vi "log analysis_gps.vi"() -> ()   [LabVIEW 2019] (continued)
22.3000,0.3276,0.3265,-0.0468,0.306680390,-0.455879554,38.607757832,0.4139,0.2956,0.5455,0.1116,0.0928,0.0789,0.2623,0.2370,5.2072,0f000001,0*4613d5e8\n\tsystem status\tnormal 2 28.100000 0 0\trobot status\t86.793506\t114.356384\t7.882400\t0.306680\t-0.455880\t51.392242\t0.481000\t-0.082000\n\t\n15:10:34.9\tlog_raw\tgps_raw\t#INSPVAXA,USB3,0,44.5,FINESTEERING,2107,281452.900,02000000,471d,15824;INS_ALIGNMENT_COMPLETE,INS_RTKFIXED,37.37116210966,126.72181674670,7.8822,22.3000,0.3215,0.3514,-0.0183,0.377751174,-0.234093113,39.308354629,0.4139,0.2956,0.5455,0.1116,0.0928,0.0789,0.2623,0.2370,5.2072,0f000001,0*f7d4e910\n\tsystem status\tnormal 2 28.100000 0 0\trobot status\t86.952206\t114.526018\t7.882200\t0.377751\t-0.234093\t50.691645\t0.575000\t0.082000\n\t\n15:10:35.4\tlog_raw\tgps_raw\t#INSPVAXA,USB3,0,49.0,FINESTEERING,2107,281453.400,02000000,471d,15824;INS_ALIGNMENT_COMPLETE,INS_RTKFIXED,37.37116361961,126.72181857489,7.8793,22.3000,0.3370,0.3634,-0.0294,0.431370913,-0.173130172,39.969478281,0.4147,0.2957,0.5475,0.1117,0.0928,0.0786,0.2622,0.2369,5.2083,0f000001,0*84da0b27\n\tsystem status\tnormal 2 28.100000 0 0\trobot status\t87.114144\t114.693597\t7.879300\t0.431371\t-0.173130\t50.030522\t0.697000\t0.271000\n\t\n15:10:35.9\tlog_raw\tgps_raw\t#INSPVAXA,USB3,0,49.0,FINESTEERING,2107,281453.900,02000000,471d,15824;INS_ALIGNMENT_COMPLETE,INS_RTKFIXED,37.37116508071,126.72182041170,7.8755,22.3000,0.3222,0.3708,0.0001,0.426257094,0.020843514,40.660737153,0.4147,0.2957,0.5475,0.1117,0.0928,0.0786,0.2622,0.2369,5.2083,0f000001,0*b9aa4650\n\tsystem status\tnormal 2 28.100000 0 0\trobot status\t87.276845\t114.855755\t7.875500\t0.426257\t0.020844\t49.339263\t0.637000\t0.224000\n\t\n15:10:36.4\tlog_raw\tgps_raw\t\tsystem status\tnormal 2 28.200000 0 0\trobot status\t87.425316\t115.004204\t7.873100\t0.306924\t-0.091173\t48.845827\t0.512000\t0.015000\n\t\n15:10:36.9\tlog_raw\tgps_raw\t\tsystem status\tnormal 2 28.200000 0 0\trobot status\t87.594195\t115.169671\t7.870000\t0.055982\t-0.430690\t48.471662\t0.488000\t0.000000\n\t\n15:10:37.4\tlog_raw\tgps_raw\t#INSPVAXA,USB3,0,47.5,FINESTEERING,2107,281455.400,02000000,471d,15824;INS_ALIGNMENT_COMPLETE,INS_RTKFIXED,37.37116944200,126.72182606901,7.8692,22.3000,0.2987,0.3736,-0.0088,0.240749777,-0.612888046,41.923306200,0.4162,0.2974,0.5511,0.1132,0.0944,0.0792,0.2618,0.2366,5.2086,0f000001,0*c27b5d3d\n\tsystem status\tnormal 2 28.200000 0 0\trobot status\t87.777961\t115.339786\t7.869200\t0.240750\t-0.612888\t48.076694\t0.495000\t0.000000\n\t\n15:10:37.9\tlog_raw\tgps_raw\t\tsystem status\tnormal 2 28.200000 0 0\trobot status\t87.930313\t115.479170\t7.868600\t0.020179\t-0.354766\t47.828050\t0.494000\t0.009000\n\t\n15:10:38.4\tlog_raw\tgps_raw\t\tsystem status\tnormal 2 28.200000 0 0\trobot status\t88.096784\t115.631090\t7.865500\t0.013870\t-0.069360\t47.540904\t0.491000\t0.018000\n\t\n15:10:38.9\tlog_raw\tgps_raw\t#INSPVAXA,USB3,0,48.0,FINESTEERING,2107,281456.900,02000000,471d,15824;INS_ALIGNMENT_COMPLETE,INS_RTKFIXED,37.37117357948,126.72183178358,7.8608,22.3000,0.3100,0.3922,-0.0117,-0.041780079,0.015103018,42.742184550,0.4159,0.2958,0.5494,0.1140,0.0949,0.0793,0.2613,0.2363,5.2090,0f000001,0*a764cc08\n\tsystem status\tnormal 2 28.200000 0 0\trobot status\t88.284148\t115.798978\t7.860800\t-0.041780\t0.015103\t47.257815\t0.495000\t0.022000\n\t\n15:10:39.4\tlog_raw\tgps_raw\t\tsystem status\tnormal 2 28.200000 0 0\trobot status\t88.440316\t115.946391\t7.860500\t-0.480884\t-0.081727\t47.108768\t0.484000\t0.025000\n\t\n15:10:39.9\tlog_raw\tgps_raw\t#INSPVAXA,USB3,0,47.5,FINESTEERING,2107,281457.900,02008000,471d,15824;INS_ALIGNMENT_COMPLETE,INS_RTKFIXED,37.37117644696,126.72183567344,7.8614,22.3000,0.3036,0.3952,-0.0191,-0.435122492,0.297928497,42.865174724,0.4156,0.2944,0.5469,0.1149,0.0954,0.0797,0.2607,0.2357,5.2097,0f000001,0*67fee73b\n\tsystem status\tnormal 2 28.200000 0 0\trobot status\t88.628705\t116.117220\t7.861400\t-0.435122\t0.297928\t47.134825\t0.508000\t0.013000\n\t\n15:10:40.4\tlog_raw\tgps_raw\t#INSPVAXA,USB3,0,48.0,FINESTEERING,2107,281458.400,02008000,471d,15824;INS_ALIGNMENT_COMPLETE,INS_RTKFIXED,37.37117789762,126.72183765812,7.8605,22.3000,0.2663,0.3794,0.0055,-0.186627591,0.430628544,42.799150387,0.4156,0.2930,0.5449,0.1157,0.0959,0.0801,0.2599,0.2351,5.2111,0f000001,0*353aab58\n\tsystem status\tnormal 2 28.200000 0 0\trobot status\t88.804505\t116.278219\t7.860500\t-0.186628\t0.430629\t47.200850\t0.465000\t0.064000\n\t\n15:10:40.9\tlog_raw\tgps_raw\t#INSPVAXA,USB3,0,48.0,FINESTEERING,2107,281458.900,02008000,471d,15824;INS_ALIGNMENT_COMPLETE,INS_RTKFIXED,37.37117931784,126.72183956069,7.8626,22.3000,0.2674,0.3686,0.0176,-0.645699086,0.378450815,42.391957050,0.4156,0.2930,0.5449,0.1157,0.0959,0.0801,0.2599,0.2351,5.2111,0f000001,0*1d8f7f17\n\tsystem status\tnormal 2 28.100000 0 0\trobot status\t88.973032\t116.435840\t7.862600\t-0.645699\t0.378451\t47.608043\t0.448000\t0.077000\n\t\n15:10:41.4\tlog_raw\tgps_raw\t\tsystem status\tnormal 2 28.000000 0 0\trobot status\t89.126711\t116.583855\t7.864100\t-0.650969\t0.083856\t48.244986\t0.484000\t0.043000\n\t\n15:10:41.9\tlog_raw\tgps_raw\t#INSPVAXA,USB3,0,50.5,FINESTEERING,2107,281459.900,02008000,471d,15824;INS_ALIGNMENT_COMPLETE,INS_RTKFIXED,37.37118223269,126.72184333763,7.8658,22.3000,0.2701,0.3610,0.0161,-0.453997018,0.223797272,40.778453294,0.4167,0.2944,0.5456,0.1164,0.0966,0.0809,0.2589,0.2343,5.2128,0f000001,0*32172057\n\tsystem status\tnormal 2 28.000000 0 0\trobot status\t89.307587\t116.759340\t7.865800\t-0.453997\t0.223797\t49.221547\t0.809000\t-0.455000\n\t\n15:10:42.4\tlog_raw\tgps_raw\t\tsystem status\tnormal 2 27.900000 0 0\trobot status\t89.451971\t116.913610\t7.868000\t-0.666596\t0.065651\t50.162265\t0.449000\t0.123000\n\t\n15:10:42.9\tlog_raw\tgps_raw\t\tsystem status\tnormal 2 28.000000 0 0\trobot status\t89.609230\t117.086793\t7.867300\t-0.761616\t0.035523\t51.116930\t0.518000\t0.000000\n\t\n15:10:43.4\tlog_raw\tgps_raw\t#INSPVAXA,USB3,0,46.5,FINESTEERING,2107,281461.400,02008000,471d,15824;INS_ALIGNMENT_COMPLETE,INS_RTKFIXED,37.37118692248,126.72184864093,7.8697,22.3000,0.3068,0.3589,-0.0063,-0.709550175,-0.051664009,37.872013250,0.4180,0.2946,0.5458,0.1159,0.0960,0.0825,0.2566,0.2324,5.2151,0f000001,0*59364c44\n\tsystem status\tnormal 2 27.900000 0 0\trobot status\t89.777344\t117.279829\t7.869700\t-0.709550\t-0.051664\t52.127987\t0.587000\t-0.105000\n\t\n15:10:43.9\tlog_raw\tgps_raw\t#INSPVAXA,USB3,0,46.5,FINESTEERING,2107,281461.900,02008000,471d,15824;INS_ALIGNMENT_COMPLETE,INS_RTKFIXED,37.37118851997,126.72185034796,7.8716,22.3000,0.2953,0.3443,0.0004,-0.635296762,0.077766272,37.199284796,0.4180,0.2946,0.5458,0.1159,0.0960,0.0825,0.2566,0.2324,5.2151,0f000001,0*e7cf6597\n\tsystem status\tnormal 2 28.100000 0 0\trobot status\t89.928550\t117.457124\t7.871600\t-0.635297\t0.077766\t52.800715\t0.554000\t-0.077000\n\t\n15:10:44.4\tlog_raw\tgps_raw\t#INSPVAXA,USB3,0,48.0,FINESTEERING,2107,281462.400,02008000,471d,15824;INS_ALIGNMENT_COMPLETE,INS_RTKFIXED,37.37119016469,126.72185198950,7.8718,22.3000,0.3140,0.3274,-0.0278,-0.753643784,0.303209826,36.783589938,0.4170,0.2921,0.5431,0.1150,0.0951,0.0832,0.2556,0.2316,5.2152,0f000001,0*71cc871c\n\tsystem status\tnormal 2 28.100000 0 0\trobot status\t90.073955\t117.639662\t7.871800\t-0.753644\t0.303210\t53.216410\t0.455000\t0.077000\n\t\n15:10:44.9\tlog_raw\tgps_raw\t#INSPVAXA,USB3,0,48.0,FINESTEERING,2107,281462.900,02008000,471d,15824;INS_ALIGNMENT_COMPLETE,INS_RTKFIXED,37.37119183431,126.72185366937,7.8730,22.3000,0.3211,0.3220,0.0114,-0.696465200,0.281664462,36.480823523,0.4170,0.2921,0.5431,0.1150,0.0951,0.0832,0.2556,0.2316,5.2152,0f000001,0*b2de4003\n\tsystem status\tnormal 2 28.100000 0 0\trobot status\t90.222755\t117.824962\t7.873000\t-0.696465\t0.281664\t53.519176\t0.660000\t-0.248000\n\t\n15:10:45.4\tlog_raw\tgps_raw\t#INSPVAXA,USB3,0,48.5,FINESTEERING,2107,281463.400,02008000,471d,15824;INS_ALIGNMENT_COMPLETE,INS_RTKFIXED,37.37119351156,126.72185532212,7.8740,22.3000,0.2696,0.3105,-0.0010,-0.845084934,0.040994289,36.443862142,0.4171,0.2926,0.5444,0.1146,0.0951,0.0842,0.2547,0.2310,5.2149,0f000001,0*1ae650cc\n\tsystem status\tnormal 2 28.100000 0 0\trobot status\t90.369153\t118.011109\t7.874000\t-0.845085\t0.040994\t53.556138\t0.360000\t0.131000\n\t\n15:10:45.9\tlog_raw\tgps_raw\t#INSPVAXA,USB3,0,48.5,FINESTEERING,2107,281463.900,02008000,471d,15824;INS_ALIGNMENT_COMPLETE,INS_RTKFIXED,37.37119483302,126.72185668642,7.8760,22.3000,0.1153,0.1917,-0.0076,-0.816856486,-0.145545038,36.378444891,0.4171,0.2926,0.5444,0.1146,0.0951,0.0842,0.2547,0.2310,5.2149,0f000001,0*1c1cdd38\n\tsystem status\tnormal 2 28.200000 0 0\trobot status\t90.490001\t118.157770\t7.876000\t-0.816856\t-0.145545\t53.621555\t0.368000\t-0.116000\n\t\n15:10:46.4\tlog_raw\tgps_raw\t#INSPVAXA,USB3,0,45.5,FINESTEERING,2107,281464.400,02000000,471d,15824;INS_ALIGNMENT_COMPLETE,INS_RTKFIXED,37.37119579175,126.72185768591,7.8792,22.3000,0.1971,0.2398,0.0010,-0.742386203,-0.127943073,36.538622941,0.4195,0.2979,0.5527,0.1161,0.0973,0.0858,0.2541,0.2308,5.2143,0f000001,0*24dc1fe0\n\tsystem status\tnormal 2 28.200000 0 0\trobot status\t90.578534\t118.264173\t7.879200\t-0.742386\t-0.127943\t53.461377\t0.317000\t-0.011000\n\t\n15:10:46.9\tlog_raw\tgps_raw\t#INSPVAXA,USB3,0,45.5,FINESTEERING,2107,281464.900,02000000,471d,15824;INS_ALIGNMENT_COMPLETE,INS_RTKFIXED,37.37119672915,126.72185869204,7.8846,22.3000,0.1715,0.2230,-0.0041,-0.675547372,-0.136073790,36.631506264,0.4195,0.2979,0.5527,0.1161,0.0973,0.0858,0.2541,0.2308,5.2143,0f000001,0*e856a3ba\n\tsystem status\tnormal 2 28.200000 0 0\trobot status\t90.667655\t118.368209\t7.884600\t-0.675547\t-0.136074\t53.368494\t0.292000\t-0.024000\n\t\n15:10:47.4\tlog_raw\tgps_raw\t#INSPVAXA,USB3,0,49.0,FINESTEERING,2107,281465.400,02000000,471d,15824;INS_ALIGNMENT_COMPLETE,INS_RTKFIXED,37.37119777976,126.72185974580,7.8895,22.3000,0.1707,0.2152,-0.0021,-0.795130387,-0.134235456,36.862190913,0.4216,0.3036,0.5603,0.1136,0.0955,0.0851,0.2538,0.2307,5.2127,0f000001,0*3dceb74e\n\tsystem status\tnormal 2 28.200000 0 0\trobot status\t90.760996\t118.484810\t7.889500\t-0.795130\t-0.134235\t53.137809\t0.295000\t-0.028000\n\t\n15:10:47.9\tlog_raw\tgps_raw\t#INSPVAXA,USB3,0,49.0,FINESTEERING,2107,281465.900,02000000,471d,15824;INS_ALIGNMENT_COMPLETE,INS_RTKFIXED,37.37119882408,126.72186080871,7.8935,22.3000,0.1975,0.2377,-0.0103,-0.927101285,0.026313679,37.093891060,0.4216,0.3036,0.5603,0.1136,0.0955,0.0851,0.2538,0.2307,5.2127,0f000001,0*b32abc1e\n\tsystem status\tnormal 2 28.200000 0 0\trobot status\t90.855146\t118.600712\t7.893500\t-0.927101\t0.026314\t52.906109\t0.296000\t-0.025000\n\t\n15:10:48.4\tlog_raw\tgps_raw\t#INSPVAXA,USB3,0,45.5,FINESTEERING,2107,281466.400,02000000,471d,15824;INS_ALIGNMENT_COMPLETE,INS_RTKFIXED,37.37119994764,126.72186191360,7.8953,22.3000,0.1896,0.2516,0.0024,-0.990040985,-0.050764765,37.290261699,0.4218,0.3053,0.5656,0.1126,0.0944,0.0842,0.2536,0.2306,5.2108,0f000001,0*ab7ec7da\n\tsystem status\tnormal 2 28.200000 0 0\trobot status\t90.953016\t118.725409\t7.895300\t-0.990041\t-0.050765\t52.709738\t0.299000\t-0.020000\n\t\n15:10:48.9\tlog_raw\tgps_raw\t#INSPVAXA,USB3,0,45.5,FINESTEERING,2107,281466.900,02000000,471d,15824;INS_ALIGNMENT_COMPLETE,INS_RTKFIXED,37.37120100149,126.72186298872,7.8973,22.3000,0.1935,0.2522,-0.0026,-0.854741520,-0.119099122,37.564308734,0.4218,0.3053,0.5656,0.1126,0.0944,0.0842,0.2536,0.2306,5.2108,0f000001,0*b7c581e3\n\tsystem status\tnormal 2 28.200000 0 0\trobot status\t91.048248\t118.842369\t7.897300\t-0.854742\t-0.119099\t52.435691\t0.315000\t-0.002000\n\t\n15:10:49.4\tlog_raw\tgps_raw\t#INSPVAXA,USB3,0,48.0,FINESTEERING,2107,281467.400,02000000,471d,15824;INS_ALIGNMENT_COMPLETE,INS_RTKFIXED,37.37120208153,126.72186408522,7.8997,22.3000,0.1778,0.2253,0.0049,-0.719912945,-0.270478243,38.035475922,0.4244,0.3113,0.5828,0.1121,0.0950,0.0843,0.2538,0.2306,5.2092,0f000001,0*8e9732d5\n\tsystem status\tnormal 2 28.200000 0 0\trobot status\t91.145374\t118.962236\t7.899700\t-0.719913\t-0.270478\t51.964524\t0.217000\t-0.146000\n\t\n15:10:49.9\tlog_raw\tgps_raw\t#INSPVAXA,USB3,0,48.0,FINESTEERING,2107,281467.900,02000000,471d,15824;INS_ALIGNMENT_COMPLETE,INS_RTKFIXED,37.37120312889,126.72186517178,7.9031,22.3000,0.2039,0.2426,0.0147,-0.720629061,-0.231870268,38.725653809,0.4244,0.3113,0.5828,0.1121,0.0950,0.0843,0.2538,0.2306,5.2092,0f000001,0*c758e7ce\n\tsystem status\tnormal 2 28.100000 0 0\trobot status\t91.241620\t119.078476\t7.903100\t-0.720629\t-0.231870\t51.274346\t0.251000\t-0.107000\n\t\n15:10:50.4\tlog_raw\tgps_raw\t#INSPVAXA,USB3,0,48.5,FINESTEERING,2107,281468.400,02000000,471d,15824;INS_ALIGNMENT_COMPLETE,INS_RTKFIXED,37.37120416086,126.72186625746,7.9066,22.3000,0.2025,0.2267,-0.0001,-0.736489084,-0.165649528,39.721937458,0.4260,0.3144,0.5975,0.1120,0.0953,0.0842,0.2539,0.2306,5.2089,0f000001,0*64b5bba4\n\tsystem status\tnormal 2 28.000000 0 0\trobot status\t91.337788\t119.193007\t7.906600\t-0.736489\t-0.165650\t50.278063\t0.273000\t-0.077000\n\t\n15:10:50.9\tlog_raw\tgps_raw\t#INSPVAXA,USB3,0,48.5,FINESTEERING,2107,281468.900,02000000,471d,15824;INS_ALIGNMENT_COMPLETE,INS_RTKFIXED,37.37120515414,126.72186733248,7.9096,22.3000,0.1860,0.2130,0.0062,-0.863833957,-0.176893088,40.861857992,0.4260,0.3144,0.5975,0.1120,0.0953,0.0842,0.2539,0.2306,5.2089,0f000001,0*48502021\n\tsystem status\tnormal 2 28.000000 0 0\trobot status\t91.433011\t119.303245\t7.909600\t-0.863834\t-0.176893\t49.138142\t0.282000\t-0.055000\n\t\n15:10:51.4\tlog_raw\tgps_raw\t#INSPVAXA,USB3,0,47.5,FINESTEERING,2107,281469.400,02000000,471d,15824;INS_ALIGNMENT_COMPLETE,INS_RTKFIXED,37.37120615783,126.72186845955,7.9127,22.3000,0.1833,0.2266,0.0157,-0.922756560,-0.128393101,41.953959499,0.4267,0.3157,0.6087,0.1119,0.0952,0.0838,0.2539,0.2306,5.2092,0f000001,0*9d6cc6cc\n\tsystem status\tnormal 2 28.000000 0 0\trobot status\t91.532845\t119.414638\t7.912700\t-0.922757\t-0.128393\t48.046041\t0.232000\t-0.142000\n\t\n15:10:51.9\tlog_raw\tgps_raw\t#INSPVAXA,USB3,0,47.5,FINESTEERING,2107,281469.900,02000000,471d,15824;INS_ALIGNMENT_COMPLETE,INS_RTKFIXED,37.37120711333,126.72186961218,7.9172,22.3000,0.1882,0.2386,0.0103,-0.812681162,-0.149481379,43.058831500,0.4267,0.3157,0.6087,0.1119,0.0952,0.0838,0.2539,0.2306,5.2092,0f000001,0*7e42c462\n\tsystem status\tnormal 2 28.000000 0 0\trobot status\t91.634943\t119.520683\t7.917200\t-0.812681\t-0.149481\t46.941169\t0.239000\t-0.134000\n\t\n15:10:52.4\tlog_raw\tgps_raw\t#INSPVAXA,USB3,0,48.0,FINESTEERING,2107,281470.400,02000000,471d,15824;INS_ALIGNMENT_COMPLETE,INS_RTKFIXED,37.37120802040,126.72187075599,7.9242,22.3000,0.1759,0.2315,0.0092,-0.712389099,-0.099720322,44.115258492,0.4228,0.3076,0.5975,0.1114,0.0938,0.0818,0.2538,0.2305,5.2102,0f000001,0*4e20fbfc\n\tsystem status\tnormal 2 28.000000 0 0\trobot status\t91.736260\t119.621353\t7.924200\t-0.712389\t-0.099720\t45.884742\t0.231000\t-0.116000\n\t\n15:10:52.9\tlog_raw\tgps_raw\t#INSPVAXA,USB3,0,48.0,FINESTEERING,2107,281470.900,02000000,471d,15824;INS_ALIGNMENT_COMPLETE,INS_RTKFIXED,37.37120891997,126.72187193685,7.9313,22.3000,0.1721,0.2325,0.0046,-0.682625247,-0.034958907,44.921832107,0.4228,0.3076,0.5975,0.1114,0.0938,0.0818,0.2538,0.2305,5.2102,0f000001,0*8a1ed08d\n\tsystem status\tnormal 2 28.100000 0 0\trobot status\t91.840859\t119.721190\t7.931300\t-0.682625\t-0.034959\t45.078168\t0.251000\t-0.082000\n\t\n15:10:53.4\tlog_raw\tgps_raw\t#INSPVAXA,USB3,0,44.5,FINESTEERING,2107,281471.400,02000000,471d,15824;INS_ALIGNMENT_COMPLETE,INS_RTKFIXED,37.37120978762,126.72187309291,7.9372,22.3000,0.1737,0.2402,0.0107,-0.896905071,0.182357572,45.734122702,0.4207,0.3039,0.5902,0.1115,0.0938,0.0806,0.2537,0.2305,5.2115,0f000001,0*f5531b04\n\tsystem status\tnormal 2 28.100000 0 0\trobot status\t91.943261\t119.817484\t7.937200\t-0.896905\t0.182358\t44.265877\t0.307000\t0.000000\n\t\n15:10:53.9\tlog_raw\tgps_raw\t#DUALANTENNAHEADINGA,USB3,0,44.5,FINESTEERING,2107,281471.900,02000000,d426,15824;SOL_COMPUTED,NARROW_FLOAT,-1.000000000,14.722629547,3.656694651,0.0,237.736404419,180.000000000,\"631T\",22,8,8,7,04,00,20,03*d908accb\n\tsystem status\tnormal 2 28.100000 0 0\trobot status\t92.048574\t119.910495\t7.943000\t-0.828598\t0.376591\t43.556063\t0.292000\t-0.018000\n\t\n15:10:54.4\tlog_raw\tgps_raw\t#INSPVAXA,USB3,0,44.5,FINESTEERING,2107,281472.400,02000000,471d,15824;INS_ALIGNMENT_COMPLETE,INS_RTKFIXED,37.37121145223,126.72187546991,7.9481,22.3000,0.1558,0.2299,0.0072,-0.729574410,0.299435928,46.987178524,0.4186,0.2997,0.5808,0.1119,0.0940,0.0794,0.2536,0.2304,5.2130,0f000001,0*ceccfdc7\n\tsystem status\tnormal 2 28.100000 0 0\trobot status\t92.153812\t120.002228\t7.948100\t-0.729574\t0.299436\t43.012821\t0.260000\t-0.072000\n\t\n15:10:54.9\tlog_raw\tgps_raw\t#DUALANTENNAHEADINGA,USB3,0,44.5,FINESTEERING,2107,281472.900,02000000,d426,15824;SOL_COMPUTED,NARROW_FLOAT,-1.000000000,19.887695313,3.310185432,0.0,262.944793701,180.000000000,\"631T\",19,8,8,7,04,00,20,03*e2f42a0a\n\tsystem status\tnormal 2 28.200000 0 0\trobot status\t92.259933\t120.093905\t7.952900\t-0.809538\t0.257343\t42.590447\t0.214000\t-0.135000\n\t\n15:10:55.4\tlog_raw\tgps_raw\t#INSPVAXA,USB3,0,47.0,FINESTEERING,2107,281473.400,02000000,471d,15824;INS_ALIGNMENT_COMPLETE,INS_RTKFIXED,37.37121309194,126.72187787297,7.9563,22.3000,0.1608,0.2402,-0.0008,-0.731141510,0.324719411,47.702294704,0.4170,0.2975,0.5726,0.1126,0.0945,0.0786,0.2534,0.2303,5.2142,0f000001,0*03d357e2\n\tsystem status\tnormal 2 28.200000 0 0\trobot status\t92.366671\t120.184208\t7.956300\t-0.731142\t0.324719\t42.297705\t0.287000\t-0.020000\n\t\n15:10:55.9\tlog_raw\tgps_raw\t#INSPVAXA,USB3,0,47.0,FINESTEERING,2107,281473.900,02000000,471d,15824;INS_ALIGNMENT_COMPLETE,INS_RTKFIXED,37.37121388735,126.72187905524,7.9593,22.3000,0.1511,0.2341,0.0050,-0.781655169,0.200652129,47.998434662,0.4170,0.2975,0.5726,0.1126,0.0945,0.0786,0.2534,0.2303,5.2142,0f000001,0*3307b87f\n\tsystem status\tnormal 2 28.200000 0 0\trobot status\t92.471394\t120.272486\t7.959300\t-0.781655\t0.200652\t42.001565\t0.293000\t-0.007000\n\t\n15:10:56.4\tlog_raw\tgps_raw\t#INSPVAXA,USB3,0,50.0,FINESTEERING,2107,281474.400,02000000,471d,15824;INS_ALIGNMENT_COMPLETE,INS_RTKFIXED,37.37121466825,126.72188022113,7.9625,22.3000,0.1592,0.2409,0.0043,-0.925136185,0.519912466,48.197361455,0.4159,0.2959,0.5651,0.1133,0.0951,0.0780,0.2531,0.2301,5.2153,0f000001,0*acbf0539\n\tsystem status\tnormal 2 28.200000 0 0\trobot status\t92.574667\t120.359152\t7.962500\t-0.925136\t0.519912\t41.802639\t0.302000\t0.000000\n\t\n15:10:56.9\tlog_raw\tgps_raw\t#DUALANTENNAHEADINGA,USB3,0,50.0,FINESTEERING,2107,281474.900,02000000,d426,15824;SOL_COMPUTED,L1_FLOAT,-1.000000000,29.703872681,-19.285949707,0.0,227.925506592,180.000000000,\"631T\",19,7,7,7,04,00,20,02*438e8014\n\tsystem status\tnormal 2 28.200000 0 0\trobot status\t92.679329\t120.444310\t7.964600\t-1.008820\t0.706696\t41.621049\t0.299000\t0.004000\n\t\n15:10:57.4\tlog_raw\tgps_raw\t#INSPVAXA,USB3,0,48.0,FINESTEERING,2107,281475.400,02000000,471d,15824;INS_ALIGNMENT_COMPLETE,INS_RTKFIXED,37.37121622258,126.72188269700,7.9646,22.3000,0.1441,0.2253,0.0054,-0.653688748,0.578968322,48.454145381,0.4152,0.2943,0.5583,0.1140,0.0955,0.0776,0.2526,0.2297,5.2166,0f000001,0*7e585380\n\tsystem status\tnormal 2 28.200000 0 0\trobot status\t92.793975\t120.531657\t7.964600\t-0.653689\t0.578968\t41.545855\t0.300000\t0.000000\n\t\n15:10:57.9\tlog_raw\tgps_raw\t#INSPVAXA,USB3,0,48.0,FINESTEERING,2107,281475.900,02000000,471d,15824;INS_ALIGNMENT_COMPLETE,INS_RTKFIXED,37.37121692154,126.72188386600,7.9655,22.3000,0.1584,0.2123,0.0124,-0.619737810,0.551987551,48.617638369,0.4152,0.2943,0.5583,0.1140,0.0955,0.0776,0.2526,0.2297,5.2166,0f000001,0*cdba2d64\n\tsystem status\tnormal 2 28.200000 0 0\trobot status\t92.897523\t120.609229\t7.965500\t-0.619738\t0.551988\t41.382362\t0.301000\t0.002000\n\t\n15:10:58.4\tlog_raw\tgps_raw\t#INSPVAXA,USB3,0,46.5,FINESTEERING,2107,281476.400,02000000,471d,15824;INS_ALIGNMENT_COMPLETE,INS_RTKFIXED,37.37121768155,126.72188507525,7.9668,22.3000,0.1354,0.2014,0.0180,-0.822035432,0.378941407,48.791141972,0.4147,0.2931,0.5519,0.1146,0.0957,0.0772,0.2519,0.2292,5.2180,0f000001,0*1e1562b5\n\tsystem status\tnormal 2 28.200000 0 0\trobot status\t93.004637\t120.693577\t7.966800\t-0.822035\t0.378941\t41.208858\t0.292000\t0.001000\n\t\n15:10:58.9\tlog_raw\tgps_raw\t#INSPVAXA,USB3,0,46.5,FINESTEERING,2107,281476.900,02000000,471d,15824;INS_ALIGNMENT_COMPLETE,INS_RTKFIXED,37.37121850161,126.72188636358,7.9688,22.3000,0.1738,0.2367,0.0108,-1.201696541,-0.232647671,48.968391321,0.4147,0.2931,0.5519,0.1146,0.0957,0.0772,0.2519,0.2292,5.2180,0f000001,0*afd5e89e\n\tsystem status\tnormal 2 28.200000 0 0\trobot status\t93.118755\t120.784590\t7.968800\t-1.201697\t-0.232648\t41.031609\t0.304000\t0.013000\n\t\n15:10:59.4\tlog_raw\tgps_raw\t#INSPVAXA,USB3,0,50.5,FINESTEERING,2107,281477.400,02000000,471d,15824;INS_ALIGNMENT_COMPLETE,INS_RTKFIXED,37.37121929078,126.72188763502,7.9707,22.3000,0.1401,0.2321,0.0104,-1.230903565,-0.339648847,49.051409136,0.4145,0.2921,0.5464,0.1152,0.0963,0.0770,0.2510,0.2285,5.2193,0f000001,0*fd6eca37\n\tsystem status\tnormal 2 28.200000 0 0\trobot status\t93.231377\t120.872175\t7.970700\t-1.230904\t-0.339649\t40.948591\t0.304000\t0.018000\n\t\n15:10:59.9\tlog_raw\tgps_raw\t#DUALANTENNAHEADINGA,USB3,0,50.5,FINESTEERING,2107,281477.900,02000000,d426,15824;SOL_COMPUTED,NARROW_FLOAT,-1.000000000,24.973518372,-6.230041504,0.0,279.644378662,180.000000000,\"631T\",18,8,8,6,04,00,20,03*2ec7f676\n\tsystem status\tnormal 2 28.200000 0 0\trobot status\t93.343059\t120.954830\t7.971600\t-1.076063\t-0.162518\t40.856489\t0.301000\t0.004000\n\t\n15:11:00.4\tlog_raw\tgps_raw\t#DUALANTENNAHEADINGA,USB3,0,45.5,FINESTEERING,2107,281478.400,02000000,d426,15824;SOL_COMPUTED,NARROW_FLOAT,-1.000000000,25.984382629,-14.421966553,0.0,321.839630127,180.000000000,\"631T\",19,7,7,6,04,00,20,03*c537a035\n\tsystem status\tnormal 2 28.200000 0 0\trobot status\t93.457296\t121.042717\t7.970400\t-1.082595\t-0.386242\t40.815336\t0.306000\t0.000000\n\t\n15:11:00.9\tlog_raw\tgps_raw\t#INSPVAXA,USB3,0,45.5,FINESTEERING,2107,281478.900,02000000,471d,15824;INS_ALIGNMENT_COMPLETE,INS_RTKFIXED,37.37122160716,126.72189152509,7.9681,22.3000,0.1537,0.2575,-0.0106,-0.771104700,-0.770425381,49.241520291,0.4142,0.2902,0.5416,0.1154,0.0959,0.0768,0.2499,0.2277,5.2192,0f000001,0*21e6a269\n\tsystem status\tnormal 2 28.200000 0 0\trobot status\t93.575953\t121.129253\t7.968100\t-0.771105\t-0.770425\t40.758480\t0.317000\t-0.004000\n\t\n15:11:01.4\tlog_raw\tgps_raw\t#INSPVAXA,USB3,0,48.0,FINESTEERING,2107,281479.400,02000000,471d,15824;INS_ALIGNMENT_COMPLETE,INS_RTKFIXED,37.37122237259,126.72189283393,7.9651,22.3000,0.1293,0.2257,0.0059,-0.612587772,-1.097823401,49.383599810,0.4139,0.2890,0.5376,0.1159,0.0956,0.0767,0.2487,0.2267,5.2174,0f000001,0*f7632e7f\n\tsystem status\tnormal 2 28.200000 0 0\trobot status\t93.691888\t121.214203\t7.965100\t-0.612588\t-1.097823\t40.616400\t0.292000\t0.007000\n\t\n15:11:01.9\tlog_raw\tgps_raw\t#INSPVAXA,USB3,0,48.0,FINESTEERING,2107,281479.900,02000000,471d,15824;INS_ALIGNMENT_COMPLETE,INS_RTKFIXED,37.37122311792,126.72189412346,7.9647,22.3000,0.1494,0.2660,0.0073,-0.587954124,-1.340332352,49.363469621,0.4139,0.2890,0.5376,0.1159,0.0956,0.0767,0.2487,0.2267,5.2174,0f000001,0*4724fb20\n\tsystem status\tnormal 2 28.200000 0 0\trobot status\t93.806112\t121.296922\t7.964700\t-0.587954\t-1.340332\t40.636530\t0.319000\t-0.007000\n\t\n15:11:02.4\tlog_raw\tgps_raw\t#DUALANTENNAHEADINGA,USB3,0,48.5,FINESTEERING,2107,281480.400,02000000,d426,15824;SOL_COMPUTED,L1_FLOAT,-1.000000000,38.387950897,-13.434600830,0.0,360.000000000,180.000000000,\"631T\",19,7,7,7,04,00,20,02*88d00c71\n\tsystem status\tnormal 2 28.200000 0 0\trobot status\t93.918035\t121.383471\t7.961400\t-0.891588\t-1.356831\t40.747449\t0.284000\t0.019000\n\t\n15:11:02.9\tlog_raw\tgps_raw\t#DUALANTENNAHEADINGA,USB3,0,48.5,FINESTEERING,2107,281480.900,02000000,d426,15824;SOL_COMPUTED,L1_FLOAT,-1.000000000,37.718753815,-13.467346191,0.0,360.000000000,180.000000000,\"631T\",19,7,7,7,04,00,20,02*9128bd3b\n\tsystem status\tnormal 2 28.200000 0 0\trobot status\t94.032799\t121.467213\t7.959200\t-0.622653\t-1.342414\t40.873530\t0.308000\t0.007000\n\t\n15:11:03.4\tlog_raw\tgps_raw\t#DUALANTENNAHEADINGA,USB3,0,46.5,FINESTEERING,2107,281481.400,02008000,d426,15824;SOL_COMPUTED,NARROW_FLOAT,-1.000000000,32.154727936,-10.026550293,0.0,255.698348999,180.000000000,\"631T\",21,8,8,7,04,00,20,03*90654ace\n\tsystem status\tnormal 2 28.200000 0 0\trobot status\t94.141894\t121.548882\t7.956300\t-0.409636\t-0.873487\t41.052834\t0.272000\t0.043000\n\t\n15:11:03.9\tlog_raw\tgps_raw\t#INSPVAXA,USB3,0,46.5,FINESTEERING,2107,281481.900,02008000,471d,15824;INS_ALIGNMENT_COMPLETE,INS_RTKFIXED,37.37122611752,126.72189916270,7.9537,22.3000,0.1376,0.2362,0.0025,-0.095529965,-0.586716272,48.576302995,0.4131,0.2860,0.5308,0.1150,0.0939,0.0764,0.2461,0.2246,5.2038,0f000001,0*d4dc6a04\n\tsystem status\tnormal 2 28.200000 0 0\trobot status\t94.252480\t121.629826\t7.953700\t-0.095530\t-0.586716\t41.423697\t0.320000\t-0.027000\n\t\n15:11:04.4\tlog_raw\tgps_raw\t#INSPVAXA,USB3,0,43.0,FINESTEERING,2107,281482.400,02008000,471d,15824;INS_ALIGNMENT_COMPLETE,INS_RTKFIXED,37.37122693129,126.72190044241,7.9507,22.3000,0.1400,0.2344,0.0009,-0.286718935,-0.542573010,48.417760410,0.4129,0.2856,0.5284,0.1143,0.0930,0.0764,0.2448,0.2237,5.1963,0f000001,0*4b0c873a\n\tsystem status\tnormal 2 28.200000 0 0\trobot status\t94.365835\t121.720141\t7.950700\t-0.286719\t-0.542573\t41.582240\t0.267000\t0.048000\n\t\n15:11:04.9\tlog_raw\tgps_raw\t#DUALANTENNAHEADINGA,USB3,0,43.0,FINESTEERING,2107,281482.900,02008000,d426,15824;SOL_COMPUTED,NARROW_FLOAT,-1.000000000,25.759243011,-24.488281250,0.0,296.027648926,180.000000000,\"631T\",21,7,7,7,04,00,20,03*7949ae50\n\tsystem status\tnormal 2 28.200000 0 0\trobot status\t94.478144\t121.806754\t7.948700\t-0.274138\t-0.373902\t41.735381\t0.350000\t-0.089000\n\t\n15:11:05.4\tlog_raw\tgps_raw\t#DUALANTENNAHEADINGA,USB3,0,49.0,FINESTEERING,2107,281483.400,02008000,d426,15824;SOL_COMPUTED,NARROW_FLOAT,-1.000000000,21.557176590,-28.431182861,0.0,309.766693115,180.000000000,\"631T\",20,8,8,7,04,00,20,03*24e13096\n\tsystem status\tnormal 2 28.200000 0 0\trobot status\t94.589326\t121.896946\t7.946400\t-0.509419\t-0.366117\t41.873006\t0.276000\t0.026000\n\t\n15:11:05.9\tlog_raw\tgps_raw\t#INSPVAXA,USB3,0,49.0,FINESTEERING,2107,281483.900,02008000,471d,15824;INS_ALIGNMENT_COMPLETE,INS_RTKFIXED,37.37122933882,126.72190424641,7.9440,22.3000,0.1298,0.2079,0.0016,-0.555050997,-0.344115137,48.037628133,0.4121,0.2847,0.5256,0.1130,0.0922,0.0763,0.2437,0.2229,5.1908,0f000001,0*4fcd94af\n\tsystem status\tnormal 2 28.200000 0 0\trobot status\t94.702787\t121.987336\t7.944000\t-0.555051\t-0.344115\t41.962372\t0.275000\t0.015000\n\t\n15:11:06.4\tlog_raw\tgps_raw\t#DUALANTENNAHEADINGA,USB3,0,50.0,FINESTEERING,2107,281484.400,02008000,d426,15824;SOL_COMPUTED,L1_FLOAT,-1.000000000,37.365016937,-21.970794678,0.0,360.000000000,180.000000000,\"631T\",19,7,7,7,04,00,20,02*e133e505\n\tsystem status\tnormal 2 28.200000 0 0\trobot status\t94.816092\t122.078802\t7.941300\t-0.509214\t-0.388195\t41.927434\t0.246000\t0.068000\n\t\n15:11:06.9\tlog_raw\tgps_raw\t#INSPVAXA,USB3,0,50.0,FINESTEERING,2107,281484.900,02008000,471d,15824;INS_ALIGNMENT_COMPLETE,INS_RTKFIXED,37.37123096597,126.72190680248,7.9384,22.3000,0.1511,0.2333,-0.0078,-0.410489938,-0.523354884,48.112153719,0.4115,0.2844,0.5237,0.1121,0.0916,0.0762,0.2426,0.2223,5.1884,0f000001,0*a1f40ef1\n\tsystem status\tnormal 2 28.200000 0 0\trobot status\t94.929199\t122.167922\t7.938400\t-0.410490\t-0.523355\t41.887846\t0.307000\t-0.014000\n\t\n15:11:07.4\tlog_raw\tgps_raw\t#DUALANTENNAHEADINGA,USB3,0,47.5,FINESTEERING,2107,281485.400,02000000,d426,15824;SOL_COMPUTED,NARROW_FLOAT,-1.000000000,34.474456787,-26.341827393,0.0,271.964752197,180.000000000,\"631T\",20,7,7,7,04,00,20,03*cc121194\n\tsystem status\tnormal 2 28.200000 0 0\trobot status\t95.038197\t122.255744\t7.935200\t-0.314008\t-0.724193\t41.803910\t0.301000\t-0.018000\n\t\n15:11:07.9\tlog_raw\tgps_raw\t#INSPVAXA,USB3,0,47.5,FINESTEERING,2107,281485.900,02000000,471d,15824;INS_ALIGNMENT_COMPLETE,INS_RTKFIXED,37.37123256957,126.72190927922,7.9317,22.3000,0.1299,0.2173,-0.0089,-0.426845608,-0.944074849,48.432879849,0.4110,0.2838,0.5218,0.1115,0.0911,0.0761,0.2417,0.2218,5.1881,0f000001,0*ee8ace9e\n\tsystem status\tnormal 2 28.200000 0 0\trobot status\t95.148585\t122.345895\t7.931700\t-0.426846\t-0.944075\t41.567120\t0.296000\t-0.027000\n\t\n15:11:08.4\tlog_raw\tgps_raw\t#DUALANTENNAHEADINGA,USB3,0,48.0,FINESTEERING,2107,281486.400,02000000,d426,15824;SOL_COMPUTED,L1_FLOAT,-1.000000000,34.864692688,-21.694915771,0.0,360.000000000,180.000000000,\"631T\",20,7,7,7,04,00,20,02*de044530\n\tsystem status\tnormal 2 28.200000 0 0\trobot status\t95.254925\t122.434334\t7.929200\t-0.583118\t-0.955090\t41.390209\t0.295000\t-0.028000\n\t\n15:11:08.9\tlog_raw\tgps_raw\t#DUALANTENNAHEADINGA,USB3,0,48.0,FINESTEERING,2107,281486.900,02000000,d426,15824;SOL_COMPUTED,L1_FLOAT,-1.000000000,35.417118073,-21.326538086,0.0,360.000000000,180.000000000,\"631T\",20,7,7,7,04,00,20,02*a4d3627b\n\tsystem status\tnormal 2 28.200000 0 0\trobot status\t95.374786\t122.532706\t7.926900\t-0.619494\t-0.937051\t41.183853\t0.303000\t-0.026000\n\t\n15:11:09.4\tlog_raw\tgps_raw\t#INSPVAXA,USB3,0,48.5,FINESTEERING,2107,281487.400,02000000,471d,15824;INS_ALIGNMENT_COMPLETE,INS_RTKFIXED,37.37123510484,126.72191313192,7.9239,22.3000,0.1508,0.2267,-0.0041,-0.710611469,-0.697297129,49.092383754,0.4097,0.2833,0.5200,0.1105,0.0907,0.0760,0.2404,0.2213,5.1897,0f000001,0*65fc2fbf\n\tsystem status\tnormal 2 28.200000 0 0\trobot status\t95.489851\t122.627267\t7.923900\t-0.710611\t-0.697297\t40.907616\t0.238000\t-0.131000\n\t\n15:11:09.9\tlog_raw\tgps_raw\t#INSPVAXA,USB3,0,48.5,FINESTEERING,2107,281487.900,02000000,471d,15824;INS_ALIGNMENT_COMPLETE,INS_RTKFIXED,37.37123588578,126.72191437981,7.9197,22.3000,0.1455,0.2377,-0.0129,-0.683157100,-0.548580830,49.602033608,0.4097,0.2833,0.5200,0.1105,0.0907,0.0760,0.2404,0.2213,5.1897,0f000001,0*fc400f11\n\tsystem status\tnormal 2 28.200000 0 0\trobot status\t95.600387\t122.713938\t7.919700\t-0.683157\t-0.548581\t40.397966\t0.257000\t-0.091000\n\t\n15:11:10.4\tlog_raw\tgps_raw\t#INSPVAXA,USB3,0,47.5,FINESTEERING,2107,281488.400,02000000,471d,15824;INS_ALIGNMENT_COMPLETE,INS_RTKFIXED,37.37123668548,126.72191567046,7.9173,22.3000,0.1286,0.2563,0.0010,-0.700638856,-0.301855154,50.490709534,0.4091,0.2828,0.5195,0.1103,0.0906,0.0760,0.2400,0.2212,5.1909,0f000001,0*20940426\n\tsystem status\tnormal 2 28.000000 0 0\trobot status\t95.714710\t122.802691\t7.917300\t-0.700639\t-0.301855\t39.509290\t0.289000\t-0.057000\n\t\n15:11:10.9\tlog_raw\tgps_raw\t#INSPVAXA,USB3,0,47.5,FINESTEERING,2107,281488.900,02000000,471d,15824;INS_ALIGNMENT_COMPLETE,INS_RTKFIXED,37.37123745255,126.72191698522,7.9152,22.3000,0.1363,0.2513,-0.0110,-0.588840465,-0.298661481,51.824057860,0.4091,0.2828,0.5195,0.1103,0.0906,0.0760,0.2400,0.2212,5.1909,0f000001,0*3253a0a6\n\tsystem status\tnormal 2 28.000000 0 0\trobot status\t95.831170\t122.887822\t7.915200\t-0.588840\t-0.298661\t38.175942\t0.297000\t-0.069000\n\t\n15:11:11.4\tlog_raw\tgps_raw\t#DUALANTENNAHEADINGA,USB3,0,48.5,FINESTEERING,2107,281489.400,02000000,d426,15824;SOL_COMPUTED,NARROW_FLOAT,-1.000000000,34.332912445,-16.076080322,0.0,273.294891357,180.000000000,\"631T\",21,7,7,7,04,00,20,02*2e8f18b8\n\tsystem status\tnormal 2 27.900000 0 0\trobot status\t95.949898\t122.972376\t7.912900\t-0.599779\t-0.338527\t36.608570\t0.233000\t-0.159000\n\t\n15:11:11.9\tlog_raw\tgps_raw\t#DUALANTENNAHEADINGA,USB3,0,48.5,FINESTEERING,2107,281489.900,02000000,d426,15824;SOL_COMPUTED,NARROW_FLOAT,-1.000000000,35.701751709,-15.985229492,0.0,272.194824219,180.000000000,\"631T\",19,7,7,7,04,00,20,03*54912f65\n\tsystem status\tnormal 2 27.900000 0 0\trobot status\t96.069390\t123.052392\t7.909700\t-0.721439\t-0.355140\t34.869410\t0.294000\t-0.053000\n\t\n15:11:12.4\tlog_raw\tgps_raw\t#DUALANTENNAHEADINGA,USB3,0,49.0,FINESTEERING,2107,281490.400,02000000,d426,15824;SOL_COMPUTED,L1_FLOAT,-1.000000000,33.157665253,-11.030181885,0.0,245.857955933,180.000000000,\"631T\",19,7,7,7,04,00,20,02*0068c7a6\n\tsystem status\tnormal 2 27.900000 0 0\trobot status\t96.191818\t123.129264\t7.907800\t-0.808399\t-0.346910\t33.250498\t0.288000\t-0.054000\n\t\n15:11:12.9\tlog_raw\tgps_raw\t#INSPVAXA,USB3,0,49.0,FINESTEERING,2107,281490.900,02000000,471d,15824;INS_ALIGNMENT_COMPLETE,INS_RTKFIXED,37.37124025850,126.72192244807,7.9063,22.3000,0.0958,0.2597,0.0085,-0.741191829,-0.240876601,58.109405467,0.4082,0.2817,0.5177,0.1106,0.0906,0.0758,0.2393,0.2210,5.1939,0f000001,0*b3d0469a\n\tsystem status\tnormal 2 27.900000 0 0\trobot status\t96.315060\t123.199234\t7.906300\t-0.741192\t-0.240877\t31.890595\t0.298000\t-0.040000\n\t\n15:11:13.4\tlog_raw\tgps_raw\t#INSPVAXA,USB3,0,49.0,FINESTEERING,2107,281491.400,02000000,471d,15824;INS_ALIGNMENT_COMPLETE,INS_RTKFIXED,37.37124087093,126.72192387521,7.9056,22.3000,0.0957,0.2456,-0.0018,-0.666118734,-0.163871029,59.496681270,0.4086,0.2815,0.5172,0.1112,0.0911,0.0758,0.2390,0.2209,5.1955,0f000001,0*877ace1f\n\tsystem status\tnormal 2 28.000000 0 0\trobot status\t96.441474\t123.267203\t7.905600\t-0.666119\t-0.163871\t30.503319\t0.304000\t-0.045000\n\t\n15:11:13.9\tlog_raw\tgps_raw\t#DUALANTENNAHEADINGA,USB3,0,49.0,FINESTEERING,2107,281491.900,02000000,d426,15824;SOL_COMPUTED,L1_FLOAT,-1.000000000,38.072498322,-12.872985840,0.0,241.422912598,180.000000000,\"631T\",19,9,9,9,04,00,20,22*0432346e\n\tsystem status\tnormal 2 28.000000 0 0\trobot status\t96.568665\t123.330118\t7.904500\t-0.611629\t-0.208521\t29.205612\t0.300000\t-0.045000\n\t\n15:11:14.4\tlog_raw\tgps_raw\t#DUALANTENNAHEADINGA,USB3,0,48.5,FINESTEERING,2107,281492.400,02000000,d426,15824;SOL_COMPUTED,L1_FLOAT,-1.000000000,43.679172516,-11.013610840,0.0,278.657897949,180.000000000,\"631T\",19,9,9,9,04,00,20,22*bdfbef21\n\tsystem status\tnormal 2 28.000000 0 0\trobot status\t96.697406\t123.389905\t7.904100\t-0.471743\t-0.224689\t28.194890\t0.305000\t-0.018000\n\t\n15:11:14.9\tlog_raw\tgps_raw\t#DUALANTENNAHEADINGA,USB3,0,48.5,FINESTEERING,2107,281492.900,02000000,d426,15824;SOL_COMPUTED,L1_FLOAT,-1.000000000,44.166721344,-11.721832275,0.0,281.896148682,180.000000000,\"631T\",20,9,9,9,04,00,20,22*48a6c000\n\tsystem status\tnormal 2 28.000000 0 0\trobot status\t96.826286\t123.446082\t7.904600\t-0.372477\t-0.149927\t27.324643\t0.365000\t0.065000\n\t\n15:11:15.4\tlog_raw\tgps_raw\t#INSPVAXA,USB3,0,42.5,FINESTEERING,2107,281493.400,02000000,471d,15824;INS_ALIGNMENT_COMPLETE,INS_RTKFIXED,37.37124296430,126.72192966667,7.9049,22.3000,0.0753,0.2701,-0.0078,-0.323936505,-0.201612973,63.426537614,0.4097,0.2821,0.5162,0.1137,0.0933,0.0757,0.2379,0.2204,5.1978,0f000001,0*1142f323\n\tsystem status\tnormal 2 28.100000 0 0\trobot status\t96.954472\t123.499529\t7.904900\t-0.323937\t-0.201613\t26.573462\t0.296000\t-0.033000\n\t\n15:11:15.9\tlog_raw\tgps_raw\t#INSPVAXA,USB3,0,42.5,FINESTEERING,2107,281493.900,02000000,471d,15824;INS_ALIGNMENT_COMPLETE,INS_RTKFIXED,37.37124340358,126.72193109595,7.9039,22.3000,0.0669,0.2621,-0.0103,-0.274820593,-0.183280206,64.003294915,0.4097,0.2821,0.5162,0.1137,0.0933,0.0757,0.2379,0.2204,5.1978,0f000001,0*917919f7\n\tsystem status\tnormal 2 28.100000 0 0\trobot status\t97.081075\t123.548281\t7.903900\t-0.274821\t-0.183280\t25.996705\t0.287000\t-0.043000\n\t\n15:11:16.4\tlog_raw\tgps_raw\t#DUALANTENNAHEADINGA,USB3,0,47.0,FINESTEERING,2107,281494.400,02000000,d426,15824;SOL_COMPUTED,L1_FLOAT,-1.000000000,39.924659729,-8.854888916,0.0,360.000000000,180.000000000,\"631T\",19,7,7,7,04,00,20,02*f82ff11c\n\tsystem status\tnormal 2 28.100000 0 0\trobot status\t97.211664\t123.598352\t7.904400\t-0.173516\t-0.210977\t25.527882\t0.231000\t-0.102000\n\t\n15:11:16.9\tlog_raw\tgps_raw\t#DUALANTENNAHEADINGA,USB3,0,47.0,FINESTEERING,2107,281494.900,02000000,d426,15824;SOL_COMPUTED,L1_FLOAT,-1.000000000,40.630737305,-7.196624756,0.0,360.000000000,180.000000000,\"631T\",19,7,7,7,04,00,20,02*f7322ed7\n\tsystem status\tnormal 2 28.100000 0 0\trobot status\t97.340068\t123.646028\t7.905000\t-0.190815\t-0.235419\t25.071870\t0.256000\t-0.075000\n\t\n15:11:17.4\tlog_raw\tgps_raw\t#DUALANTENNAHEADINGA,USB3,0,52.0,FINESTEERING,2107,281495.400,02000000,d426,15824;SOL_COMPUTED,L1_FLOAT,-1.000000000,40.645214081,-8.830108643,0.0,360.000000000,180.000000000,\"631T\",18,7,7,7,04,00,20,02*8609447b\n\tsystem status\tnormal 2 28.200000 0 0\trobot status\t97.470080\t123.694067\t7.905000\t-0.125585\t-0.333623\t24.668388\t0.408000\t0.158000\n\t\n15:11:17.9\tlog_raw\tgps_raw\t#INSPVAXA,USB3,0,52.0,FINESTEERING,2107,281495.900,02000000,471d,15824;INS_ALIGNMENT_COMPLETE,INS_RTKFIXED,37.37124512541,126.72193695200,7.9047,22.3000,0.0463,0.2469,-0.0072,0.000083390,-0.348047959,65.534193450,0.4125,0.2835,0.5158,0.1165,0.0957,0.0756,0.2356,0.2190,5.1978,0f000001,0*14e6bfac\n\tsystem status\tnormal 2 28.200000 0 0\trobot status\t97.599794\t123.739371\t7.904700\t8.339000E-5\t-0.348048\t24.465807\t0.267000\t-0.061000\n\t\n15:11:18.4\tlog_raw\tgps_raw\t#DUALANTENNAHEADINGA,USB3,0,49.0,FINESTEERING,2107,281496.400,02000000,d426,15824;SOL_COMPUTED,NARROW_FLOAT,-1.000000000,36.124023438,-7.202545166,0.0,327.448486328,180.000000000,\"631T\",21,7,7,7,04,00,20,03*2df9ffe6\n\tsystem status\tnormal 2 28.200000 0 0\trobot status\t97.726631\t123.783734\t7.904200\t-0.058576\t-0.411548\t24.254597\t0.294000\t-0.010000\n\t\n15:11:18.9\tlog_raw\tgps_raw\t#DUALANTENNAHEADINGA,USB3,0,49.0,FINESTEERING,2107,281496.900,02000000,d426,15824;SOL_COMPUTED,NARROW_FLOAT,-1.000000000,36.800415039,-8.357086182,0.0,335.148284912,180.000000000,\"631T\",21,7,7,7,04,00,20,03*89694ba0\n\tsystem status\tnormal 2 28.200000 0 0\trobot status\t97.857023\t123.827865\t7.902700\t-0.090473\t-0.381739\t24.045732\t0.290000\t-0.006000\n\t\n15:11:19.4\tlog_raw\tgps_raw\t#DUALANTENNAHEADINGA,USB3,0,45.5,FINESTEERING,2107,281497.400,02000000,d426,15824;SOL_COMPUTED,NARROW_FLOAT,-1.000000000,35.379425049,-14.173278809,0.0,252.907455444,180.000000000,\"631T\",20,8,8,7,04,00,20,03*7b0cb3e2\n\tsystem status\tnormal 2 28.200000 0 0\trobot status\t97.988469\t123.873077\t7.902000\t-0.155451\t-0.327488\t23.836141\t0.289000\t-0.006000\n\t\n15:11:19.9\tlog_raw\tgps_raw\t#DUALANTENNAHEADINGA,USB3,0,45.5,FINESTEERING,2107,281497.900,02000000,d426,15824;SOL_COMPUTED,NARROW_FLOAT,-1.000000000,35.681621552,-15.419891357,0.0,255.079315186,180.000000000,\"631T\",18,8,8,7,04,00,20,03*3e48e9bf\n\tsystem status\tnormal 2 28.200000 0 0\trobot status\t98.118399\t123.914958\t7.902100\t-0.109922\t-0.275380\t23.671221\t0.300000\t-0.004000\n\t\n15:11:20.4\tlog_raw\tgps_raw\t#DUALANTENNAHEADINGA,USB3,0,47.0,FINESTEERING,2107,281498.400,02008000,d426,15824;SOL_COMPUTED,L1_FLOAT,-1.000000000,40.500751495,-12.284759521,0.0,360.000000000,180.000000000,\"631T\",19,7,7,7,04,00,20,02*8d7c2d6f\n\tsystem status\tnormal 2 28.200000 0 0\trobot status\t98.250192\t123.959125\t7.901500\t-0.037488\t-0.243011\t23.485467\t0.296000\t0.000000\n\t\n15:11:20.9\tlog_raw\tgps_raw\t\tsystem status\tnormal 2 28.200000 0 0\trobot status\t98.384075\t124.002284\t7.901600\t0.025329\t-0.306954\t23.281238\t0.303000\t0.000000\n\t\n15:11:21.4\tlog_raw\tgps_raw\t#DUALANTENNAHEADINGA,USB3,0,46.5,FINESTEERING,2107,281499.400,02008000,d426,15824;SOL_COMPUTED,L1_FLOAT,-1.000000000,47.084907532,-15.694274902,0.0,360.000000000,180.000000000,\"631T\",19,7,7,7,04,00,20,02*f0de5a60\n\tsystem status\tnormal 2 28.200000 0 0\trobot status\t98.514050\t124.046709\t7.902400\t-0.087568\t-0.323192\t23.084948\t0.294000\t-0.003000\n\t\n15:11:21.9\tlog_raw\tgps_raw\t#DUALANTENNAHEADINGA,USB3,0,46.5,FINESTEERING,2107,281499.900,02008000,d426,15824;SOL_COMPUTED,L1_FLOAT,-1.000000000,46.870197296,-16.724273682,0.0,360.000000000,180.000000000,\"631T\",18,7,7,7,04,00,20,02*32f34491\n\tsystem status\tnormal 2 28.200000 0 0\t
